vi "littleEndianFlatten.vi"() -> (2 "data string":string)   [LabVIEW 2016]
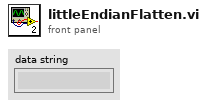
[diagram p1: front panel]
types:
  T1 = enum16{"big-endian, network order", "native, host order", "little-endian"}
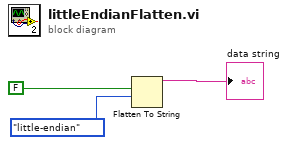
[diagram p0: block diagram]
diagram:
  n1 = Flatten To String(prepend array or string size? (T)=FALSE, byte order (0:big-endian, network order)=T1."little-endian") -> (anything=w1:cluster{}, data string=→"data string":string)  [unwired: 1 in, 2 out]
